vi "Configure 8 Input Logic Operation Input.vi"(6 "Selected Function (1)":u8=1 min=1 max=2, 7 "Unit Address (1)":u8=1, 8 "error in (no error)":errorcluster, 9 "Input Value (0)":i32, 10 "Selected Input (1)":u8=1 min=1 max=8, 11 "VISA resource name":refnum<visa-resource-name>) -> (0 "error out":errorcluster, 3 "VISA resource name out":refnum<visa-resource-name>)   [LabVIEW 2014, in "Eurotherm 35xx Series.lvlib"]
doc: "This VI sets the input values for the Eight Input Logic Operation Function."
uses:
  <instrlib>/Eurotherm 35xx Series/Eurotherm 35xx Series.lvlib
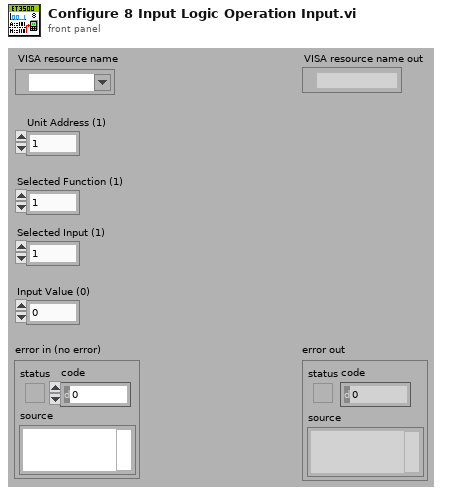
[diagram p1: front panel]
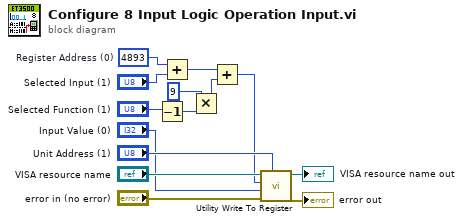
[diagram p0: block diagram]
diagram:
  w3 = 4893  # Register Address (0)
  n1 = Decrement(x="Selected Function (1)") -> (x-1=w8:u8)
  n2 = Add(x=w3, y="Selected Input (1)") -> (x+y=w1:i32)
  n3 = Multiply(x=u8 9, y=w8) -> (x*y=w6:u8)
  n4 = Add(x=w1, y=w6) -> (x+y=w5:i32)
  n5 = call <instrlib>:"Utility Write To Register.vi"("Unit Address (1)"="Unit Address (1)", "error in (no error)"="error in (no error)", "Data (0)"="Input Value (0)", "Register Address (0)"=w5, "VISA resource name"="VISA resource name") -> ("error out"=→"error out":errorcluster, "VISA resource name out"=→"VISA resource name out":refnum<visa-resource-name>)  [unwired: 5 in]
